vi "Create_Empty_Rx_Channels.vi"(8 "Nb Channels":i32=16, 11 "Rx Channels In":T1[](array[typedef])=[{"Labels Settings"=[], "channel handle"=0, "channel #"=0}, {"Labels Settings"=[], "channel handle"=0, "channel #"=0}, {"Labels Settings"=[], "channel handle"=0, "channel #"=0}, {"Labels Settings"=[], "channel handle"=0, "channel #"=0}] {"Labels Settings"."Label Timestamp Channel Data Reference" format="%.0x"; "Labels Settings"."Label Disable/Trigger Channel Reference" format="%.0x"; "Labels Settings"."Word"."Param Setting"."Item Refs" format="%.0x"; "Labels Settings"."Word"."Param Setting"."Num Bits" min=1 max=32; "Labels Settings"."Word"."Param Setting"."Start Bit" min=8 max=31; "Labels Settings"."Label" format="%.0o"}) -> (3 "Rx Channels Out":T1[](array[typedef])=[{"Labels Settings"=[{"Name"="label 1", "xmlName"="100", "Label"=23, "transferPeriod"=0, "SDI_Enabled"=FALSE, "SDI"=0, "Word"={"Param Setting"={"Start Bit"=[], "Num Bits"=[], "Signed?"=[], "ScaleFac"=[], "ScaleOffset"=[], "Block Data Refs"=[], "Encoding"=[], "Values Array"=[], "Item Refs"=[]}}, "TransferType"=enum."ScheduledLabel", "has timestamp?"=TRUE, "Label Disable/Trigger Channel Reference"=18446744073709551615, "Message Handle"=0, "Initialized?"=FALSE, "Word Initial Raw Value"=0, "Label Timestamp Channel Data Reference"=0}, {"Name"="label 2", "xmlName"="200", "Label"=24, "transferPeriod"=0, "SDI_Enabled"=FALSE, "SDI"=0, "Word"={"Param Setting"={"Start Bit"=[], "Num Bits"=[], "Signed?"=[], "ScaleFac"=[], "ScaleOffset"=[], "Block Data Refs"=[], "Encoding"=[], "Values Array"=[], "Item Refs"=[]}}, "TransferType"=enum."ScheduledLabel", "has timestamp?"=TRUE, "Label Disable/Trigger Channel Reference"=18446744073709551615, "Message Handle"=0, "Initialized?"=FALSE, "Word Initial Raw Value"=0, "Label Timestamp Channel Data Reference"=0}, {"Name"="label 3", "xmlName"="300", "Label"=25, "transferPeriod"=0, "SDI_Enabled"=FALSE, "SDI"=0, "Word"={"Param Setting"={"Start Bit"=[], "Num Bits"=[], "Signed?"=[], "ScaleFac"=[], "ScaleOffset"=[], "Block Data Refs"=[], "Encoding"=[], "Values Array"=[], "Item Refs"=[]}}, "TransferType"=enum."ScheduledLabel", "has timestamp?"=TRUE, "Label Disable/Trigger Channel Reference"=18446744073709551615, "Message Handle"=0, "Initialized?"=FALSE, "Word Initial Raw Value"=0, "Label Timestamp Channel Data Reference"=0}, {"Name"="label 4", "xmlName"="400", "Label"=26, "transferPeriod"=0, "SDI_Enabled"=FALSE, "SDI"=0, "Word"={"Param Setting"={"Start Bit"=[], "Num Bits"=[], "Signed?"=[], "ScaleFac"=[], "ScaleOffset"=[], "Block Data Refs"=[], "Encoding"=[], "Values Array"=[], "Item Refs"=[]}}, "TransferType"=enum."ScheduledLabel", "has timestamp?"=TRUE, "Label Disable/Trigger Channel Reference"=18446744073709551615, "Message Handle"=0, "Initialized?"=FALSE, "Word Initial Raw Value"=0, "Label Timestamp Channel Data Reference"=0}], "channel handle"=0, "channel #"=0}, {"Labels Settings"=[{"Name"="label 1", "xmlName"="101", "Label"=23, "transferPeriod"=0, "SDI_Enabled"=FALSE, "SDI"=0, "Word"={"Param Setting"={"Start Bit"=[], "Num Bits"=[], "Signed?"=[], "ScaleFac"=[], "ScaleOffset"=[], "Block Data Refs"=[], "Encoding"=[], "Values Array"=[], "Item Refs"=[]}}, "TransferType"=enum."ScheduledLabel", "has timestamp?"=TRUE, "Label Disable/Trigger Channel Reference"=18446744073709551615, "Message Handle"=0, "Initialized?"=FALSE, "Word Initial Raw Value"=0, "Label Timestamp Channel Data Reference"=0}, {"Name"="label 2", "xmlName"="201", "Label"=24, "transferPeriod"=0, "SDI_Enabled"=FALSE, "SDI"=0, "Word"={"Param Setting"={"Start Bit"=[], "Num Bits"=[], "Signed?"=[], "ScaleFac"=[], "ScaleOffset"=[], "Block Data Refs"=[], "Encoding"=[], "Values Array"=[], "Item Refs"=[]}}, "TransferType"=enum."ScheduledLabel", "has timestamp?"=TRUE, "Label Disable/Trigger Channel Reference"=18446744073709551615, "Message Handle"=0, "Initialized?"=FALSE, "Word Initial Raw Value"=0, "Label Timestamp Channel Data Reference"=0}, {"Name"="label 3", "xmlName"="301", "Label"=25, "transferPeriod"=0, "SDI_Enabled"=FALSE, "SDI"=0, "Word"={"Param Setting"={"Start Bit"=[], "Num Bits"=[], "Signed?"=[], "ScaleFac"=[], "ScaleOffset"=[], "Block Data Refs"=[], "Encoding"=[], "Values Array"=[], "Item Refs"=[]}}, "TransferType"=enum."ScheduledLabel", "has timestamp?"=TRUE, "Label Disable/Trigger Channel Reference"=18446744073709551615, "Message Handle"=0, "Initialized?"=FALSE, "Word Initial Raw Value"=0, "Label Timestamp Channel Data Reference"=0}, {"Name"="label 4", "xmlName"="401", "Label"=26, "transferPeriod"=0, "SDI_Enabled"=FALSE, "SDI"=0, "Word"={"Param Setting"={"Start Bit"=[], "Num Bits"=[], "Signed?"=[], "ScaleFac"=[], "ScaleOffset"=[], "Block Data Refs"=[], "Encoding"=[], "Values Array"=[], "Item Refs"=[]}}, "TransferType"=enum."ScheduledLabel", "has timestamp?"=TRUE, "Label Disable/Trigger Channel Reference"=18446744073709551615, "Message Handle"=0, "Initialized?"=FALSE, "Word Initial Raw Value"=0, "Label Timestamp Channel Data Reference"=0}, {"Name"="label 5", "xmlName"="501", "Label"=27, "transferPeriod"=0, "SDI_Enabled"=FALSE, "SDI"=0, "Word"={"Param Setting"={"Start Bit"=[], "Num Bits"=[], "Signed?"=[], "ScaleFac"=[], "ScaleOffset"=[], "Block Data Refs"=[], "Encoding"=[], "Values Array"=[], "Item Refs"=[]}}, "TransferType"=enum."ScheduledLabel", "has timestamp?"=TRUE, "Label Disable/Trigger Channel Reference"=18446744073709551615, "Message Handle"=0, "Initialized?"=FALSE, "Word Initial Raw Value"=0, "Label Timestamp Channel Data Reference"=0}, {"Name"="label 6", "xmlName"="601", "Label"=28, "transferPeriod"=0, "SDI_Enabled"=FALSE, "SDI"=0, "Word"={"Param Setting"={"Start Bit"=[], "Num Bits"=[], "Signed?"=[], "ScaleFac"=[], "ScaleOffset"=[], "Block Data Refs"=[], "Encoding"=[], "Values Array"=[], "Item Refs"=[]}}, "TransferType"=enum."ScheduledLabel", "has timestamp?"=TRUE, "Label Disable/Trigger Channel Reference"=18446744073709551615, "Message Handle"=0, "Initialized?"=FALSE, "Word Initial Raw Value"=0, "Label Timestamp Channel Data Reference"=0}], "channel handle"=0, "channel #"=1}, {"Labels Settings"=[{"Name"="label 1", "xmlName"="102", "Label"=23, "transferPeriod"=0, "SDI_Enabled"=FALSE, "SDI"=0, "Word"={"Param Setting"={"Start Bit"=[], "Num Bits"=[], "Signed?"=[], "ScaleFac"=[], "ScaleOffset"=[], "Block Data Refs"=[], "Encoding"=[], "Values Array"=[], "Item Refs"=[]}}, "TransferType"=enum."ScheduledLabel", "has timestamp?"=TRUE, "Label Disable/Trigger Channel Reference"=18446744073709551615, "Message Handle"=0, "Initialized?"=FALSE, "Word Initial Raw Value"=0, "Label Timestamp Channel Data Reference"=0}, {"Name"="label 2", "xmlName"="202", "Label"=24, "transferPeriod"=0, "SDI_Enabled"=FALSE, "SDI"=0, "Word"={"Param Setting"={"Start Bit"=[], "Num Bits"=[], "Signed?"=[], "ScaleFac"=[], "ScaleOffset"=[], "Block Data Refs"=[], "Encoding"=[], "Values Array"=[], "Item Refs"=[]}}, "TransferType"=enum."ScheduledLabel", "has timestamp?"=TRUE, "Label Disable/Trigger Channel Reference"=18446744073709551615, "Message Handle"=0, "Initialized?"=FALSE, "Word Initial Raw Value"=0, "Label Timestamp Channel Data Reference"=0}, {"Name"="label 3", "xmlName"="302", "Label"=25, "transferPeriod"=0, "SDI_Enabled"=FALSE, "SDI"=0, "Word"={"Param Setting"={"Start Bit"=[], "Num Bits"=[], "Signed?"=[], "ScaleFac"=[], "ScaleOffset"=[], "Block Data Refs"=[], "Encoding"=[], "Values Array"=[], "Item Refs"=[]}}, "TransferType"=enum."ScheduledLabel", "has timestamp?"=TRUE, "Label Disable/Trigger Channel Reference"=18446744073709551615, "Message Handle"=0, "Initialized?"=FALSE, "Word Initial Raw Value"=0, "Label Timestamp Channel Data Reference"=0}, {"Name"="label 4", "xmlName"="402", "Label"=26, "transferPeriod"=0, "SDI_Enabled"=FALSE, "SDI"=0, "Word"={"Param Setting"={"Start Bit"=[], "Num Bits"=[], "Signed?"=[], "ScaleFac"=[], "ScaleOffset"=[], "Block Data Refs"=[], "Encoding"=[], "Values Array"=[], "Item Refs"=[]}}, "TransferType"=enum."ScheduledLabel", "has timestamp?"=TRUE, "Label Disable/Trigger Channel Reference"=18446744073709551615, "Message Handle"=0, "Initialized?"=FALSE, "Word Initial Raw Value"=0, "Label Timestamp Channel Data Reference"=0}, {"Name"="label 5", "xmlName"="502", "Label"=27, "transferPeriod"=0, "SDI_Enabled"=FALSE, "SDI"=0, "Word"={"Param Setting"={"Start Bit"=[], "Num Bits"=[], "Signed?"=[], "ScaleFac"=[], "ScaleOffset"=[], "Block Data Refs"=[], "Encoding"=[], "Values Array"=[], "Item Refs"=[]}}, "TransferType"=enum."ScheduledLabel", "has timestamp?"=TRUE, "Label Disable/Trigger Channel Reference"=18446744073709551615, "Message Handle"=0, "Initialized?"=FALSE, "Word Initial Raw Value"=0, "Label Timestamp Channel Data Reference"=0}, {"Name"="label 6", "xmlName"="602", "Label"=28, "transferPeriod"=0, "SDI_Enabled"=FALSE, "SDI"=0, "Word"={"Param Setting"={"Start Bit"=[], "Num Bits"=[], "Signed?"=[], "ScaleFac"=[], "ScaleOffset"=[], "Block Data Refs"=[], "Encoding"=[], "Values Array"=[], "Item Refs"=[]}}, "TransferType"=enum."ScheduledLabel", "has timestamp?"=TRUE, "Label Disable/Trigger Channel Reference"=18446744073709551615, "Message Handle"=0, "Initialized?"=FALSE, "Word Initial Raw Value"=0, "Label Timestamp Channel Data Reference"=0}, {"Name"="label 7", "xmlName"="702", "Label"=29, "transferPeriod"=0, "SDI_Enabled"=FALSE, "SDI"=0, "Word"={"Param Setting"={"Start Bit"=[], "Num Bits"=[], "Signed?"=[], "ScaleFac"=[], "ScaleOffset"=[], "Block Data Refs"=[], "Encoding"=[], "Values Array"=[], "Item Refs"=[]}}, "TransferType"=enum."ScheduledLabel", "has timestamp?"=TRUE, "Label Disable/Trigger Channel Reference"=18446744073709551615, "Message Handle"=0, "Initialized?"=FALSE, "Word Initial Raw Value"=0, "Label Timestamp Channel Data Reference"=0}, {"Name"="label 8", "xmlName"="802", "Label"=30, "transferPeriod"=0, "SDI_Enabled"=FALSE, "SDI"=0, "Word"={"Param Setting"={"Start Bit"=[], "Num Bits"=[], "Signed?"=[], "ScaleFac"=[], "ScaleOffset"=[], "Block Data Refs"=[], "Encoding"=[], "Values Array"=[], "Item Refs"=[]}}, "TransferType"=enum."ScheduledLabel", "has timestamp?"=TRUE, "Label Disable/Trigger Channel Reference"=18446744073709551615, "Message Handle"=0, "Initialized?"=FALSE, "Word Initial Raw Value"=0, "Label Timestamp Channel Data Reference"=0}], "channel handle"=0, "channel #"=2}, {"Labels Settings"=[{"Name"="label 1 SDI 01", "xmlName"="10301", "Label"=23, "transferPeriod"=0, "SDI_Enabled"=TRUE, "SDI"=1, "Word"={"Param Setting"={"Start Bit"=[], "Num Bits"=[], "Signed?"=[], "ScaleFac"=[], "ScaleOffset"=[], "Block Data Refs"=[], "Encoding"=[], "Values Array"=[], "Item Refs"=[]}}, "TransferType"=enum."ScheduledLabel", "has timestamp?"=TRUE, "Label Disable/Trigger Channel Reference"=18446744073709551615, "Message Handle"=0, "Initialized?"=FALSE, "Word Initial Raw Value"=0, "Label Timestamp Channel Data Reference"=0}, {"Name"="label 1 SDI 10", "xmlName"="10310", "Label"=23, "transferPeriod"=0, "SDI_Enabled"=TRUE, "SDI"=10, "Word"={"Param Setting"={"Start Bit"=[], "Num Bits"=[], "Signed?"=[], "ScaleFac"=[], "ScaleOffset"=[], "Block Data Refs"=[], "Encoding"=[], "Values Array"=[], "Item Refs"=[]}}, "TransferType"=enum."ScheduledLabel", "has timestamp?"=TRUE, "Label Disable/Trigger Channel Reference"=18446744073709551615, "Message Handle"=0, "Initialized?"=FALSE, "Word Initial Raw Value"=0, "Label Timestamp Channel Data Reference"=0}, {"Name"="label 2", "xmlName"="203", "Label"=24, "transferPeriod"=0, "SDI_Enabled"=FALSE, "SDI"=0, "Word"={"Param Setting"={"Start Bit"=[], "Num Bits"=[], "Signed?"=[], "ScaleFac"=[], "ScaleOffset"=[], "Block Data Refs"=[], "Encoding"=[], "Values Array"=[], "Item Refs"=[]}}, "TransferType"=enum."ScheduledLabel", "has timestamp?"=TRUE, "Label Disable/Trigger Channel Reference"=18446744073709551615, "Message Handle"=0, "Initialized?"=FALSE, "Word Initial Raw Value"=0, "Label Timestamp Channel Data Reference"=0}], "channel handle"=0, "channel #"=3}] {"Labels Settings"."Label Timestamp Channel Data Reference" format="%.0x"; "Labels Settings"."Label Disable/Trigger Channel Reference" format="%.0x"; "Labels Settings"."Word"."Param Setting"."Item Refs" format="%.0x"; "Labels Settings"."Word"."Param Setting"."Num Bits" min=1 max=32; "Labels Settings"."Word"."Param Setting"."Start Bit" min=8 max=31; "Labels Settings"."Label" format="%.0o"})   [LabVIEW 2020, in "Ballard Arinc-429 Engine.lvlib"]
doc: "We allocate memory space for all Channels even if not used. Goal is to ensure we don't allocate memory once running."
uses:
  Ballard Arinc-429 Engine.lvlib
  Shared/Controls and Global/RT HW Channel.ctl
  Shared/Controls and Global/RT Label Settings.ctl
  Shared/Controls and Global/Label.ctl
  Shared/Controls and Global/transferPeriod.ctl
  Shared/Controls and Global/RT Word Settings.ctl
  Shared/Controls and Global/RT Param Setting.ctl
  Shared/Controls and Global/Start Bit.ctl
  Shared/Controls and Global/Number of Bits.ctl
  <vilib>/NI VeriStand/Custom Device API/Block Data Reference.ctl
  <vilib>/NI VeriStand/Custom Device API/Data Reference.ctl
  <vilib>/NI VeriStand/Custom Device API/Custom Device Item Ref.ctl
  Shared/Controls and Global/TransferType.ctl
  Shared/Ballard Arinc-429 Shared.lvlib
  <vilib>/NI VeriStand/Custom Device API/Custom Device API.lvlib
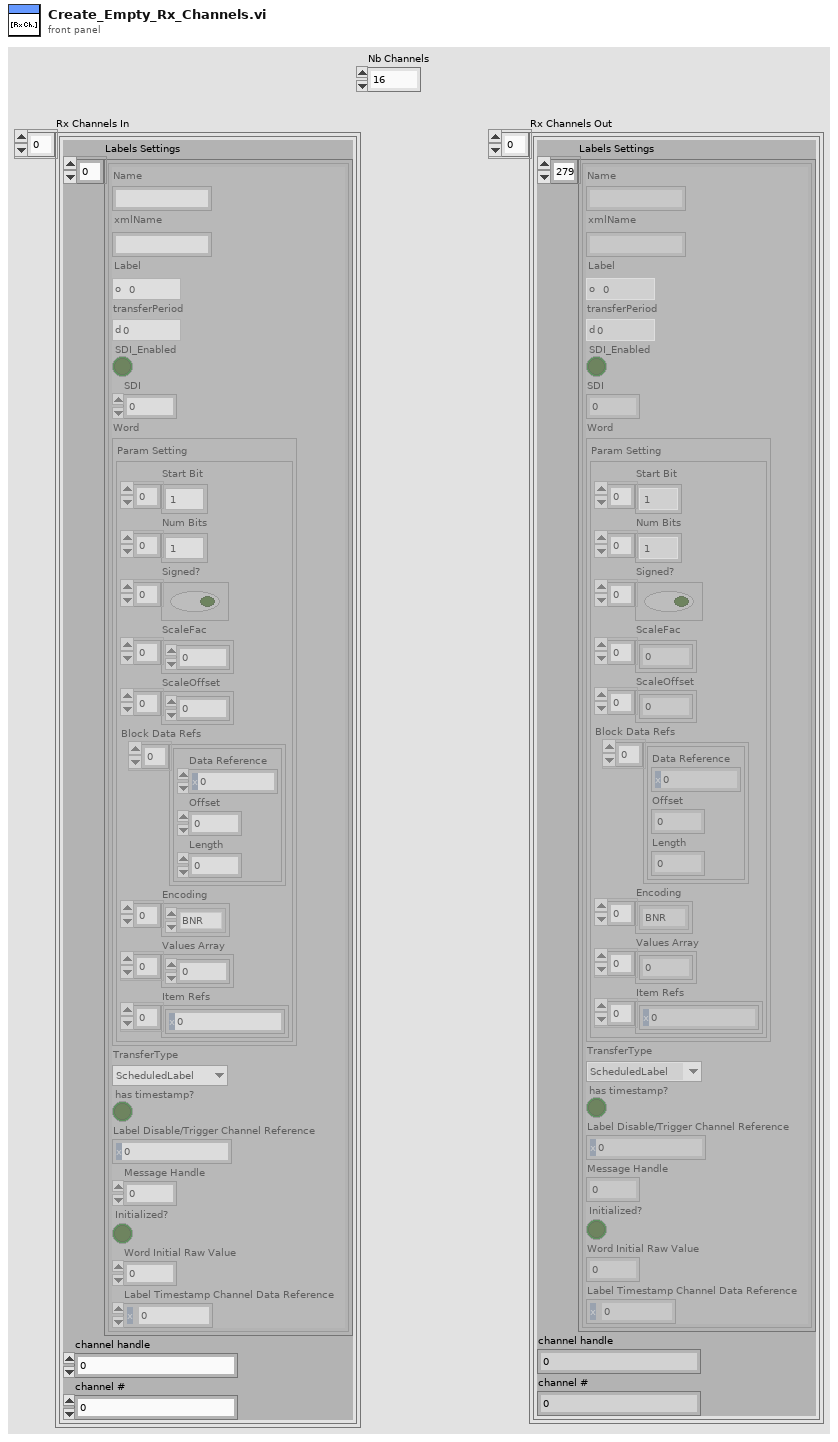
[diagram p1: front panel]
types:
  T1 = typedef "Ballard Arinc-429 Shared.lvlib/RT HW Channel.ctl" = cluster{"Labels Settings":T2[], "channel handle":u64, "channel #":u16}
  T2 = typedef "Ballard Arinc-429 Shared.lvlib/RT Label Settings.ctl" = cluster{"Name":string, "xmlName":string, "Label":T3, "transferPeriod":T4, "SDI_Enabled":bool, "SDI":u8, "Word":T5, "TransferType":T12, "has timestamp?":bool, "Label Disable/Trigger Channel Reference":T11, "Message Handle":u64, "Initialized?":bool, "Word Initial Raw Value":u32, "Label Timestamp Channel Data Reference":T10}
  T3 = typedef "Ballard Arinc-429 Shared.lvlib/Label.ctl" = u8
  T4 = typedef "Ballard Arinc-429 Shared.lvlib/transferPeriod.ctl" = u32
  T5 = typedef "Ballard Arinc-429 Shared.lvlib/RT Word Settings.ctl" = cluster{"Param Setting":T6}
  T6 = typedef "Ballard Arinc-429 Shared.lvlib/RT Param Setting.ctl" = cluster{"Start Bit":T7[], "Num Bits":T8[], "Signed?":bool[], "ScaleFac":dbl[], "ScaleOffset":dbl[], "Block Data Refs":T9[], "Encoding":enum16{"BNR", "BCD", "Discrete"}[], "Values Array":dbl[], "Item Refs":T11[]}
  T7 = typedef "Ballard Arinc-429 Shared.lvlib/Start Bit.ctl" = i32
  T8 = typedef "Ballard Arinc-429 Shared.lvlib/Number of Bits.ctl" = i32
  T9 = typedef "Custom Device API.lvlib/Block Data Reference.ctl" = cluster{"Data Reference":T10, "Offset":u64, "Length":u64}
  T10 = typedef "Custom Device API.lvlib/Data Reference.ctl" = i32
  T11 = typedef "Custom Device API.lvlib/Custom Device Item Ref.ctl" = u64
  T12 = typedef "Ballard Arinc-429 Shared.lvlib/TransferType.ctl" = enum16{"ScheduledLabel", "Acyclic", "Block", "Strobe"}
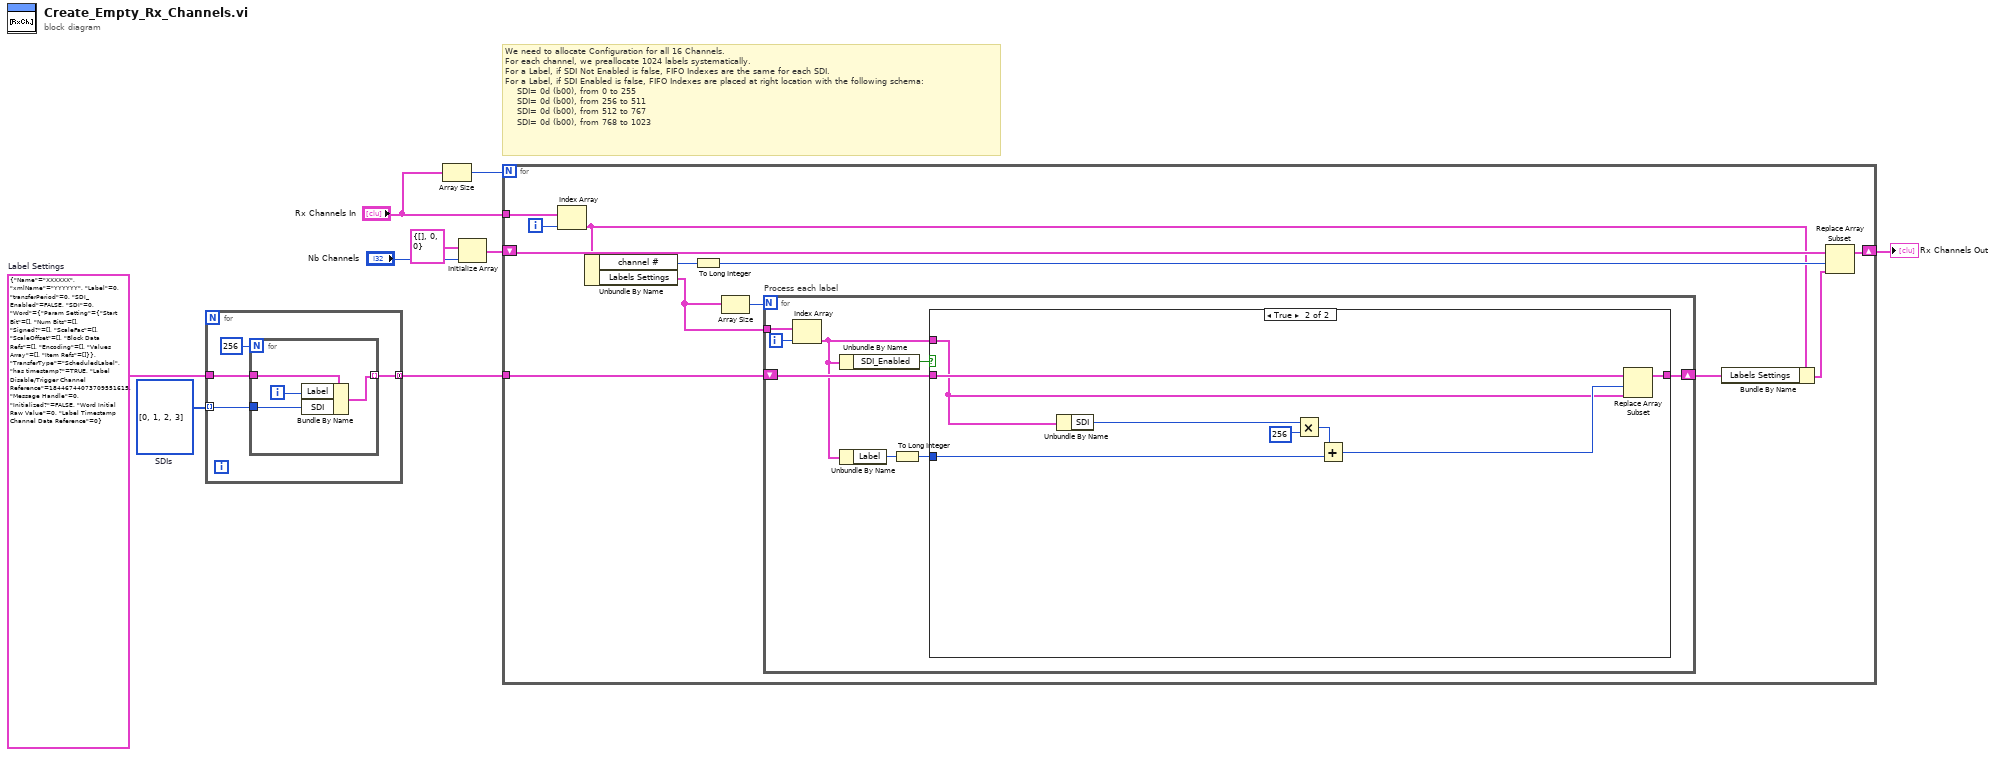
[diagram p0: block diagram]
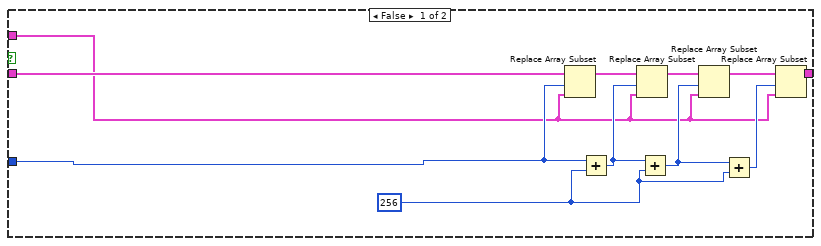
[diagram p2: hidden frame]
diagram:
  w3 = u8[] [0, 1, 2, 3]  # SDIs
  w4 = T2 {"Name"="XXXXXX", "xmlName"="YYYYYY", "Label"=0, "transferPeriod"=0, "SDI_Enabled"=FALSE, "SDI"=0, "Word"={"Param Setting"={"Start Bit"=[], "Num Bits"=[], "Signed?"=[], "ScaleFac"=[], "ScaleOffset"=[], "Block Data Refs"=[], "Encoding"=[], "Values Array"=[], "Item Refs"=[]}}, "TransferType"=enum."ScheduledLabel", "has timestamp?"=TRUE, "Label Disable/Trigger Channel Reference"=18446744073709551615, "Message Handle"=0, "Initialized?"=FALSE, "Word Initial Raw Value"=0, "Label Timestamp Channel Data Reference"=0}  # Label Settings
  # "We need to allocate Configuration for all 16 Channels.\nFor each channel, we preallocate 1024 labels systematically.\nFor a Label, if SDI Not Enabled is false, FIFO Indexes are the same for each SDI.\nFor a Label, if SDI Enabled is false, FIFO Indexes are placed at right location with the following schema:\n    SDI= 0d (b00), from 0 to 255\n    SDI= 0d (b00), from 256 to 511\n    SDI= 0d (b00), from 512 to 767\n    SDI= 0d (b00), from 768 to 1023"
  n1 = for {
    tunnel: w4 -> [w12]
    tunnel: [w11] -> w2 mode=concatenating
    tunnel: w3 -> [w10] mode=indexing
    n2 = for {
      N: 256 -> [_]
      tunnel: w12 -> [w17]
      tunnel: [w15] -> w11 mode=indexing
      tunnel: w10 -> [w14]
      i -> [w16]
      n3 = Bundle By Name(cluster=w17, "Label"=w16, "SDI"=w14) -> (w15:T2)
    }
  }
  n4 = Array Size(array="Rx Channels In") -> (size(s)=w6:i32)
  n5 = Initialize Array(T1 {"Labels Settings"=[], "channel handle"=0, "channel #"=0} ("HW Channel"), "Nb Channels") -> (w7:T1[])
  n6 = for {
    N: w6 -> [_]
    shift-right: [w27] -> w1
    shift-left: w7 -> [w28]
    tunnel: "Rx Channels In" -> [w26]
    tunnel: w2 -> [w23]
    i -> [w29]
    n7 = Index Array(array=w26, index=w29) -> (element=w20:T1)
    n8 = Unbundle By Name(w20) -> ("channel #"=w25:u16, "Labels Settings"=w22:T2[])
    n9 = To Long Integer(number=w25) -> (32bit integer=w24:i32)
    n10 = Array Size(array=w22) -> (size(s)=w21:i32)
    n11 = for "Process each label" {
      N: w21 -> [_]
      tunnel: w22 -> [w35]
      shift-right: [w30] -> w19
      shift-left: w23 -> [w36]
      i -> [w34]
      n12 = Index Array(array=w35, index=w34) -> (element=w33:T2)
      n13 = Unbundle By Name(w33) -> ("SDI_Enabled"=w37:bool)
      n14 = Unbundle By Name(w33) -> ("Label"=w32:T3)
      n15 = To Long Integer(number=w32) -> (32bit integer=w31:i32)
      n16 = case shown="True" w37 {
        tunnel: w36 -> [w48 w54]
        tunnel: w33 -> [w38 w49]
        tunnel: w31 -> [w39 w53]
        tunnel: [w40 w52] -> w30
        frame False {
          w43 = 256 ("y")
          n17 = Replace Array Subset(array=w48, new element=w38, index=w39) -> (w47:T2[])
          n18 = Add(x=w39, y=w43) -> (x+y=w46:i32)
          n19 = Replace Array Subset(array=w47, new element=w38, index=w46) -> (w45:T2[])
          n20 = Add(x=w46, y=w43) -> (x+y=w44:i32)
          n21 = Replace Array Subset(array=w45, new element=w38, index=w44) -> (w41:T2[])
          n22 = Add(x=w44, y=w43) -> (x+y=w42:i32)
          n23 = Replace Array Subset(array=w41, new element=w38, index=w42) -> (w40:T2[])
        }
        frame True {
          n24 = Unbundle By Name(w49) -> ("SDI"=w51:u8)
          n25 = Multiply(x=w51, y=256) -> (x*y=w55:i32)
          n26 = Add(x=w55, y=w53) -> (x+y=w50:i32)
          n27 = Replace Array Subset(array=w54, new element=w49, index=w50) -> (w52:T2[])
        }
      }
    }
    n28 = Bundle By Name(cluster=w20, "Labels Settings"=w19) -> (w18:T1)
    n29 = Replace Array Subset(array=w28, new element=w18, index=w24) -> (w27:T1[])
  }
  "Rx Channels Out" <- w1
